vi "Delay Complete.vi"(8 "error in (no error)":errorcluster, 11 "Idle in":refnum<class "Idle.lvclass">) -> (0 "error out":errorcluster, 3 "State Actor out":refnum<class "State Actor.lvclass">)   [LabVIEW 2024, in "Sample State Actor.lvlib" / "Idle.lvclass"]
uses:
  Idle.lvclass
  State Actor/State Actor.lvclass
  Active/Active.lvclass
  C:/Users/ottoa/OneDrive/Desktop/working copies/stateActor/src/State Actor/State Actor.lvclass
  Idle.lvclass/Idle.ctl
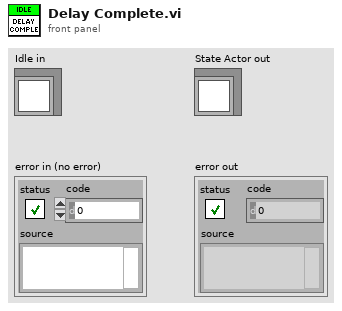
[diagram p1: front panel]
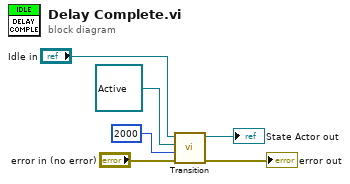
[diagram p0: block diagram]
diagram:
  n1 = call-dynamic "Transition.vi"("error in (no error)"="error in (no error)", "Milliseconds To Wait (-1, forever)"=2000, "Target State Actor in"=refnum<class "Active.lvclass"> refnum ("Sample State Actor.lvlib:Active.lvclass"), "State Actor in"="Idle in") -> ("error out"=→"error out":errorcluster, "State Actor out"=→"State Actor out":refnum<class "State Actor.lvclass">)  [unwired: 6 in]
